vi "毕设初次修改版.vi"() -> ()   [LabVIEW 2018]
uses:
  <vilib>/addons/control/pid/pid.llb/PID (DBL).vi
  <vilib>/express/express arith-compare/Formula/XNode/ExpressFormulaBlockNode.xnode
  <vilib>/addons/control/pid/NI_PID_pid.lvlib
panel:
  out "密码文件路径":path
  out "操作人员0+密码":string[][](array[string])
  out "管理人员1+密码":string[][](array[string])
  out "用户名的顺序":u16
  out "用户类别":u8
  out "Error Out":errorcluster caption="错误输出"
  in  "Error In":errorcluster caption="错误输入"
  out "选项卡":T1(tab)
  in  "进入":bool
  in  "实验三界面":bool
  in  "其他界面":bool
  in  "实验二界面":bool
  in  "实验一界面":bool
  in  "提交界面":bool
  in  "公告栏":string[](array[string])=["欢迎您试用本实验平台", "本次的实验内容有", "1xxxxxxxx", "2cccccccc", "3dddddd", "4xxxxxxxx", "5vvvvvvvv"]
  in  "退出":bool
  out "图片":picture caption="新图片"
  in  "用户管理":bool
  out "当前用户类别":string
  out "当前用户名":string
  out "时间":string
  out "小卡":enum32{"1.1", "1.2"}(tab)
  in  "下页":bool
  out "过程变量和设定值":cluster{dbl, "SP：":dbl}(graph)
  out "操作变量":dbl(graph)
  out "MV：":dbl(slide) scale=-100.0..100.0
  in  "SP：":dbl(slide) min=0.0 max=0.0 scale=0.0..120.0
  out "PV：":dbl(slide) scale=0.0..120.0
  in  "PID增益设定":T2={"比例增益(Kc)"=1.0, "积分时间(Ti，分)"=0.002, "微分时间(Td，分)"=0.002} {"微分时间(Td，分)" format="%.3f"; "积分时间(Ti，分)" format="%.3f"; "比例增益(Kc)" format="%.3f"}
  in  "实验一开始":bool
  in  "实验一暂停":bool
  in  "返回 2":bool
  out "实验1图":dbl[](graph)
  in  "上页":bool
  out "动态性能指标显示":T3
  out "是否合格显示":T4
  out "尝试次数":string
  out "可否提交":bool
  in  "返回 3":bool
  out "上升时间":dbl
  out "调节时间":dbl
  out "超调量":dbl
  in  "实验二暂停":bool
  in  "实验二开始":bool
  in  "对象特性设置":cluster{"num":dbl[], "den":dbl[]}={"num"=[1.0], "den"=[0.02, 1.0]}
  in  "PID增益设置":cluster{"Kp":dbl, "Ki":dbl, "Kd":dbl}={"Kp"=1.5, "Ki"=0.35, "Kd"=1.0}
  out "XY图":cluster{dbl[], dbl[]}(graph)
  in  "SP":dbl(slide) min=0.0 max=0.0 scale=0.0..120.0
  in  "返回 4":bool
  in  "Word保存地址":path=path "F:/LabVIEW练习/毕设/实验报告.doc"
  in  "提交确定":bool
  in  "学号:":string
  in  "姓名:":string="小明"
  in  "ExcelS.path":path=path "F:/LabVIEW练习/毕设/实验成绩.xls" caption="Excel保存路径"
  in  "空白":bool
  in  "初始化":bool
  in  "返回":bool
  in  "Excel模板路径":path=path "F:/LabVIEW练习/毕设/实验成绩.xls"
  in  "Word模板路径":path=path "F:/LabVIEW练习/毕设/实验报告模板.doc"
  out "实验3图表":dbl(graph)
  in  "实验三暂停":bool
  in  "实验三开始":bool
  in  "返回 5":bool
  in  "Kp":dbl=30.0 format="%#_13g"
  out "source":string
  out "尝试次数":u32
  in  "超限累计":i32
  out "数组":dbl[](array[numeric])=[0.15946790534816901, 0.35556228083290553, 0.5907826417638008, 0.8494826417638008, 1.1081826417638008, 1.3668826417638007, 1.6255826417638006, 1.8842826417638006, 2.1429826417638007, 2.401682641763801, 2.660382641763801, 2.919082641763801, 3.1777826417638013, 3.4364826417638015, 3.6951826417638016, 3.9538826417638018, 4.2125826417638015, 4.471282641763802, 4.729982641763802, 4.988682641763802, 5.247382641763802, 5.506082641763802, 5.764782641763802, 6.0234826417638025, 6.282182641763803, 6.540882641763803, 6.799582641763803, 7.058282641763803, 7.316982641763803, 7.5756826417638035, 7.834382641763804, 8.093082641763804, 8.351782641763803, 8.610482641763802, 8.869182641763802, 9.1278826417638, 9.3865826417638, 9.6452826417638, 9.903982641763799, 10.162682641763798, 10.421382641763797, 10.680082641763796, 10.938782641763796, 11.197482641763795, 11.456182641763794, 11.714882641763793, 11.973582641763793, 12.232282641763792, 12.490982641763791, 12.74968264176379, 13.00838264176379, 13.267082641763789, 13.525782641763788, 13.784482641763788, 14.043182641763787, 14.301882641763786, 14.560582641763785, 14.819282641763785, 15.077982641763784, 15.336682641763783, 15.595382641763782, 15.854082641763782, 16.112782641763783, 16.371482641763784, 16.630182641763785, 16.888882641763786, 17.147582641763787, 17.406282641763788, 17.66498264176379, 17.92368264176379, 18.18238264176379, 18.441082641763792, 18.699782641763793, 18.958482641763794, 19.217182641763795, 19.475882641763796, 19.734582641763797, 19.9932826417638, 20.2519826417638, 20.5106826417638, 20.7693826417638, 21.028082641763802, 21.286782641763804, 21.545482641763805, 21.804182641763806, 22.062882641763807, 22.321582641763808, 22.58028264176381, 22.83898264176381, 23.09768264176381, 23.356382641763812, 23.615082641763813, 23.873782641763814, 24.132482641763815, 24.391182641763816, 24.649882641763817, 24.908582641763818, 25.16728264176382, 25.42598264176382, 25.68468264176382, 25.943382641763822, 26.202082641763823, 26.460782641763824, 26.719482641763825, 26.978182641763826, 27.236882641763827, 27.49558264176383, 27.75428264176383, 28.01298264176383, 28.27168264176383, 28.530382641763833, 28.789082641763834, 29.047782641763835, 29.306482641763836, 29.565182641763837, 29.823882641763838, 30.08258264176384, 30.34128264176384, 30.59998264176384, 30.858682641763842, 31.117382641763843, 31.376082641763844, 31.634782641763845, 31.893482641763846, 32.152182641763844, 32.41088264176384, 32.66958264176384, 32.928282641763836, 33.186982641763834, 33.44568264176383, 33.70438264176383, 33.963082641763826, 34.221782641763824, 34.48048264176382, 34.73918264176382, 34.997882641763816, 35.25658264176381, 35.51528264176381, 35.77372176165425, 36.031884459742486, 36.289771162313485, 36.54738216334767, 36.80471775760098, 37.061778239505244, 37.318522130243544, 37.57467358720941, 37.8299594264456, 38.084107940043786, 38.33686499688974, 38.587925999781845, 38.837015689907915, 39.08390098833731, 39.32828579607282, 39.56990831464298, 39.80852799499046, 40.04390159016064, 40.275777925533525, 40.503874950422215, 40.72793097876865, 40.94778181593828, 41.16322788169536, 41.3740472034328, 41.580023389427126, 41.78087973060037, 41.97645279482925, 42.166568681508785, 42.35103471778728, 42.52957941340393, 42.70208708634859, 42.86840732714809, 43.02827548540423, 43.18150954430742, 43.32806311134, 43.46781164646614, 43.600619222636375, 43.726357743660884, 43.84490694692867, 43.956154516980234, 44.05986646431542, 44.15606406402364, 44.24453639469577, 44.32519057948923, 44.39795443410196, 44.462764470554774, 44.51956602229976, 44.5684623722877, 44.60942425329443, 44.64227082069252, 44.666977641637374, 44.683534283119904, 44.69193920908696, 44.692359011378294, 44.68465028908381, 44.668999121914815, 44.64527563307593, 44.61352408042584, 44.57379545987751, 44.52614939302406, 44.47081710257968, 44.407867701626955, 44.3372216673248, 44.25897957356577, 44.17340367346343, 44.0804305099236, 43.98034675420013, 43.87326265304072, 43.75930728668722, 43.63846143518952, 43.511038790252734, 43.377022593732704, 43.23673818240778, 43.09033207622225, 42.93782851259838, 42.77956724262933, 42.615570642290564, 42.44618643585735, 42.271586813576505, 42.091838302223536, 41.90729733314443, 41.71802441898804, 41.52425881526584, 41.32633897695649, 41.12446160950261, 40.918741029655656, 40.70954089926177, 40.4969648106794, 40.281375841949064, 40.06298482798073, 39.84203160577297, 39.61875810290718, 39.39332769049512, 39.166094497507856, 38.937206459131936, 38.707011747084934, 38.47566953230472, 38.24346340376417, 38.01064870010497, 37.7774810808516, 37.54421607075162, 37.31114593136907, 37.07849129310784, 36.84650071747841, 36.615378575927984, 36.38537198581724, 36.156943040417275, 35.93015564000529, 35.70525048381508, 35.482464651506554, 35.26203247520919, 35.04418528714419, 34.82918977838842, 34.61728362150174, 34.40866418976721, 34.203545417677866, 34.002152710466156, 33.80468049370989, 33.611355630079316, 33.42235243373588, 33.237840660649525, 33.058071096130554, 32.88318656057269, 32.71334221077529, 32.548785239587595, 32.38970558748683, 32.23635039277429, 32.0887213027308, 31.94692772347299, 31.811109866020686, 31.681500382105583, 31.558141994624826, 31.441138071257893, 31.330710906159855, 31.226982177337977, 31.130051544807788, 31.03989192894575, 30.956574187060063, 30.880298416516695, 30.811016574667573, 30.748779172798816, 30.693770570174408, 30.64604383266606, 30.605500125335514, 30.57216235661245, 30.546191212341355, 30.52746301020953, 30.515979813151755, 30.511739148217686, 30.514730768837623, 30.525082405205367, 30.54262096493095, 30.567314262688704, 30.599121227790977, 30.63799326089107, 30.684022094229924, 30.737138109376353, 30.79712134083411, 30.864047204647928, 30.937674402846334, 31.01791864742922, 31.104680413124612, 31.197997533983642, 31.297601112667355, 31.403524770877823, 31.51548742435686, 31.633369889626856, 31.75717052786516, 31.886727545997974, 32.02188775690319, 32.16249207258547, 32.30824736260859, 32.45925547191968, 32.615179595589765, 32.77573670801291, 32.940882235017824, 33.110406544352976, 33.28411560358437, 33.46181107958789, 33.64318536552284, 33.82805847807178, 34.01632346763871, 34.20774500171118, 34.40210761886112, 34.59910568351407, 34.79863001296244, 35.00043309118822, 35.20421455937076, 35.409776861426906, 35.616895997678924, 35.82540967343328, 36.03500330478898, 36.245529997989294, 36.45673189274724, 36.66833177613277, 36.88016878368664, 37.09198479004521, 37.30354852280296, 37.514602306871495, 37.72494707482634, 37.93437652215988, 38.142624707699454, 38.349505294607624, 38.5547654289942, 38.758213276831206, 38.95961027411947, 39.15877000170116, 39.355468869927705, 39.54949168753746, 39.74066037677261, 39.92877582472998, 40.11361003289667, 40.29498171485171, 40.47268498177152, 40.64651067819616, 40.816326941874074, 40.98192711472907, 41.14317621204567, 41.29986838770229, 41.451821738844906, 41.5988799580375, 41.7409664432832, 41.87795719408764, 42.0097157520009, 42.13611165526278, 42.257020452567055, 42.372232010346224, 42.481617154649165, 42.585166458979025, 42.6826931531345, 42.774090098791774, 42.859376819902224, 42.938376129353465, 43.0110039302606, 43.0773083298165, 43.13700634690593, 43.19026686553209, 43.23706044447938, 43.27722730725126, 43.310855788692564, 43.33780207941015, 43.35817371768441, 43.37183675931807, 43.37878738416311, 43.379031648389216, 43.372714902851996, 43.35985733742113, 43.340486081998, 43.31463518904689, 43.28234558282003, 43.2436650014862, 43.198513698357374, 43.14695891512083, 43.08906997124019, 43.024922996561216, 42.95460080492671, 42.878324985411076, 42.79604942541201, 42.708016010792086, 42.61432063883826, 42.51494734919351, 42.41015434896103, 42.299927660461705, 42.184411727942404, 42.06386503485702, 41.938293151587985, 41.80785840805722, 41.672713132822174, 41.53312773424592, 41.389244209130915, 41.241117376020824, 41.08893540101152, 40.932975542979875, 40.77329393535387, 40.61018892311368, 40.44382249205406, 40.27428885036583, 40.10180013164225, 39.926634944570246, 39.74896521510243, 39.568986518363765, 39.38689637097467, 39.20289414894689, 39.017114489970886, 38.82984923352281, 38.641279065899965, 38.45160880070593, 38.2609929339156, 38.06966498568467, 37.87787826534298, 37.68577681806894]
  # "结果显示"
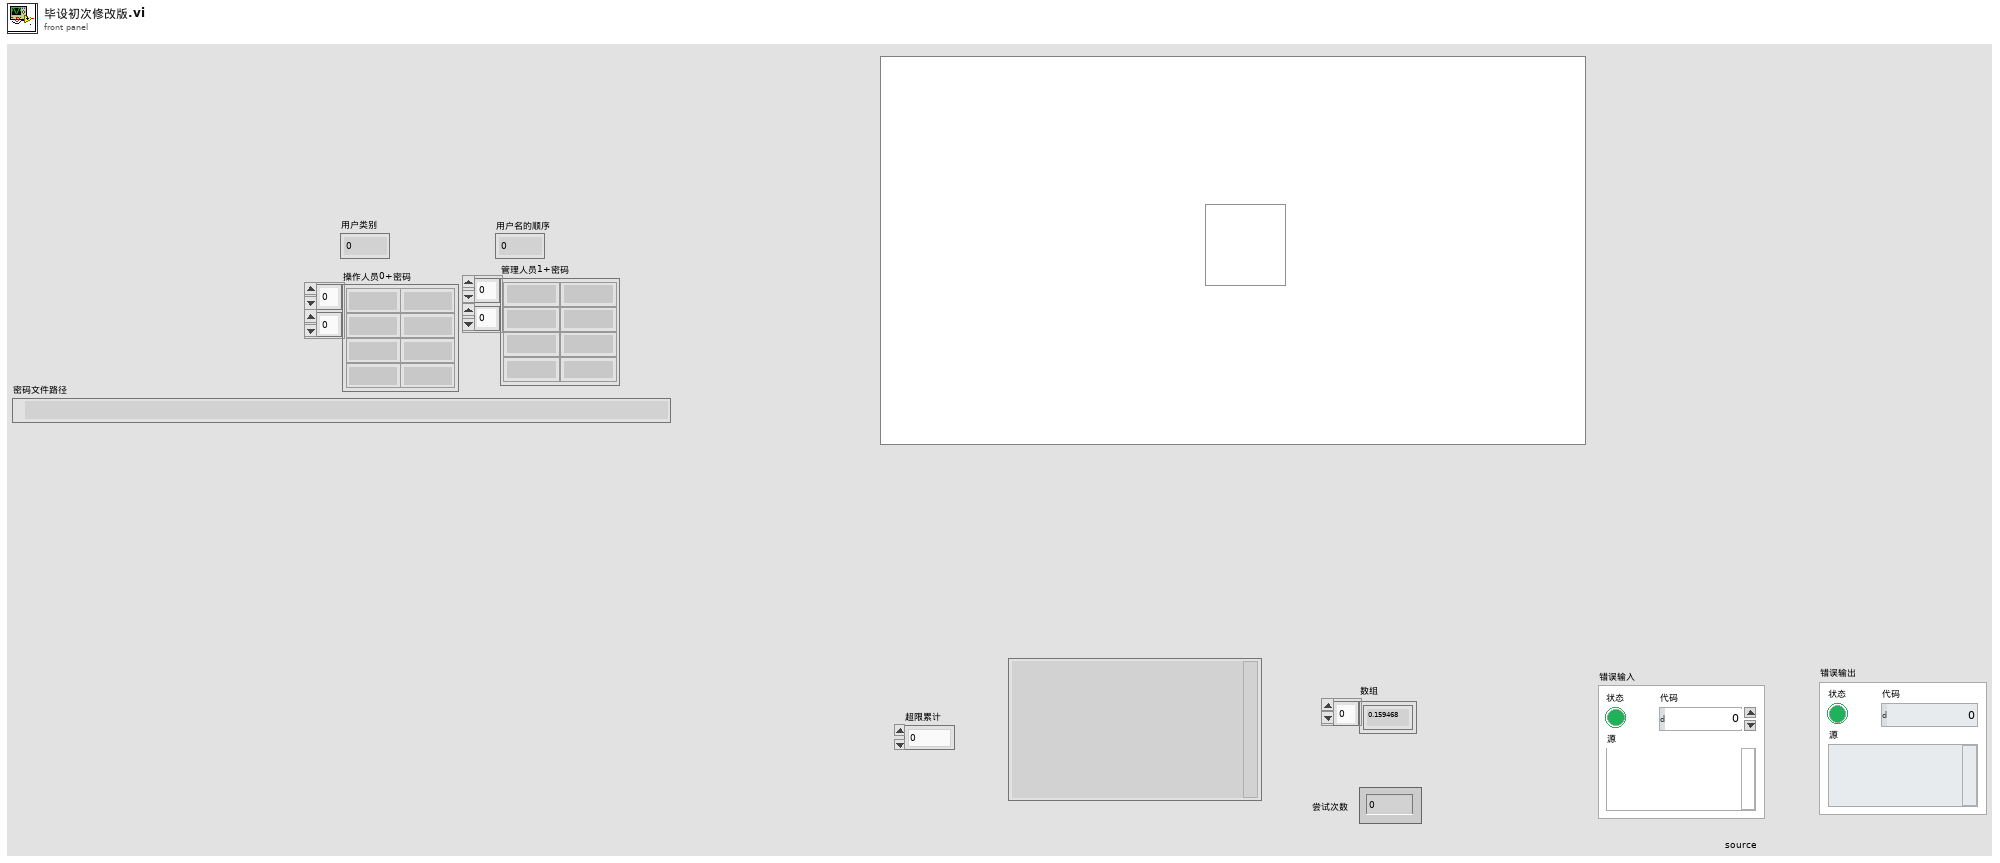
[diagram p1: front panel]
types:
  T1 = enum32{"登录", "公告", "实验1", "实验2", "提交", "其他", "实验3"}
  T2 = cluster{"比例增益(Kc)":dbl, "积分时间(Ti，分)":dbl, "微分时间(Td，分)":dbl}
  T3 = cluster{"超调量":string, "振荡频率":string, "调节时间":string, " 峰值时间":string, "阻尼比 ":string}
  T4 = cluster{"超调量":string, "振荡频率":string, "调节时间":string}
  T5 = typedef "全局事件选择.ctl" = enum16{"初始化", "等待操作", "空白", "退出", "进入", "提交确定", "返回主界面", "实验一界面", "实验二界面", "提交界面", "实验二开始", "实验一开始", "实验一暂停", "其他界面", "实验三界面", "实验三开始", "实验二暂停", "实验三暂停", "用户管理"}
  T6 = cluster{"操作人员0+密码":string[][], "管理人员1+密码":string[][]}
  T7 = enum32{"invalid app kind", "Development System", "Run Time System", "Student Edition", "Embedded LabVIEW", "Evaluation", "Custom"}
  T8 = cluster{"Excel模板路径":path, "Word模板路径":path, "ExcelS.path":path, "Word保存地址":path}
  T9 = cluster{"Font Name:":string, "Size":i16, "Strikeout?":bool, "Italic?":bool, bool, "Outline?":bool, "Shadow?":bool, "Bold?":bool}
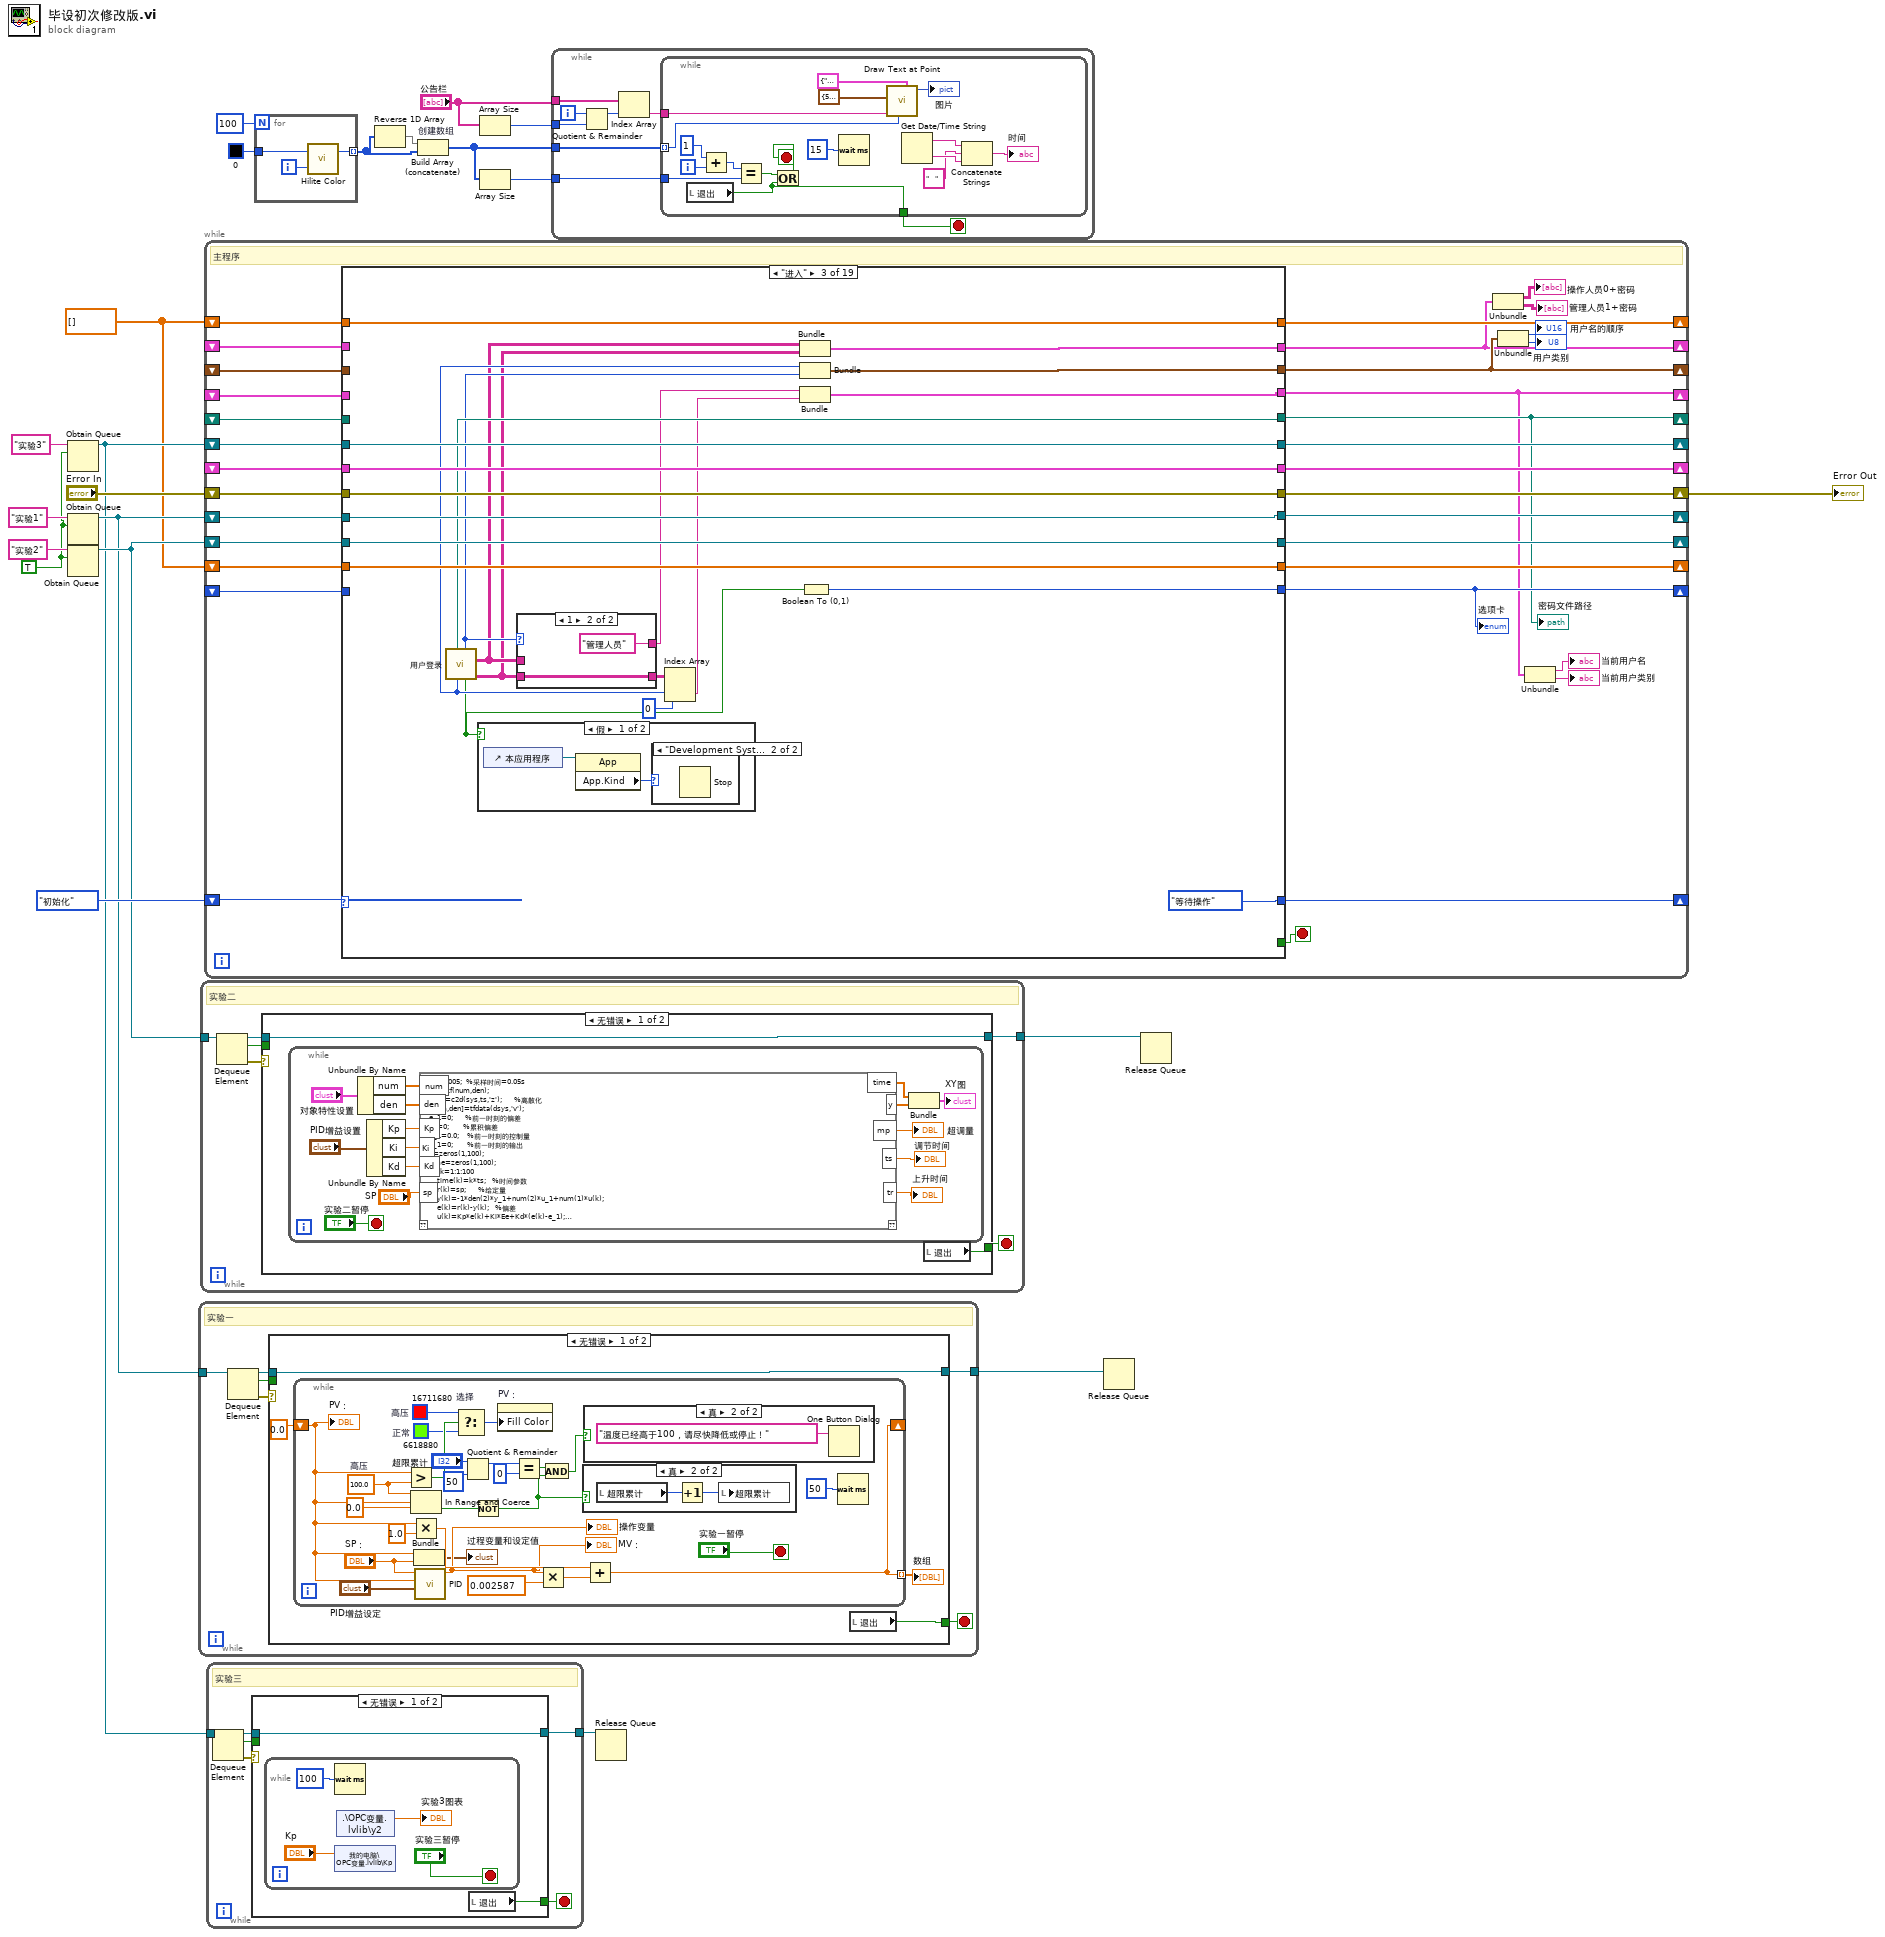
[diagram p0: block diagram]
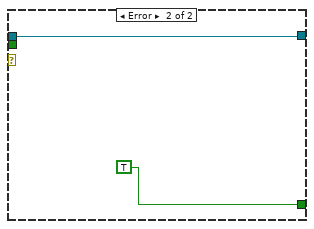
[diagram p2: hidden frame]
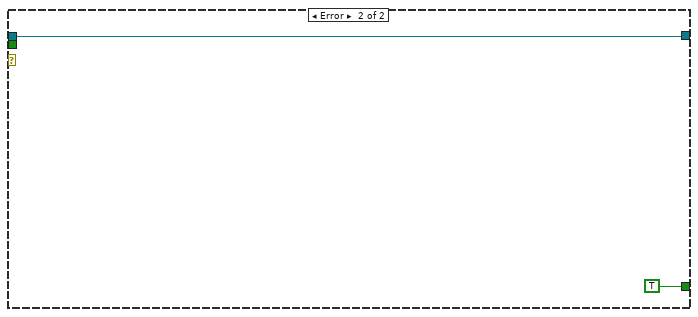
[diagram p5: hidden frame]
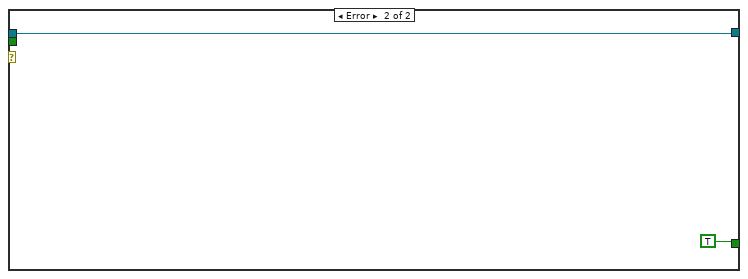
[diagram p6: hidden frame]
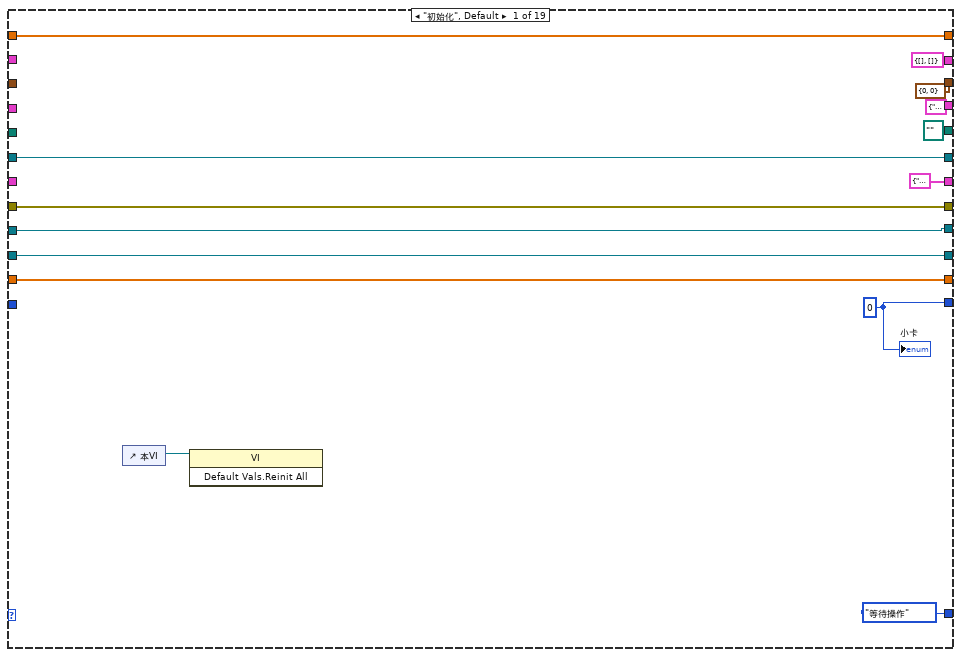
[diagram p7: hidden frame]
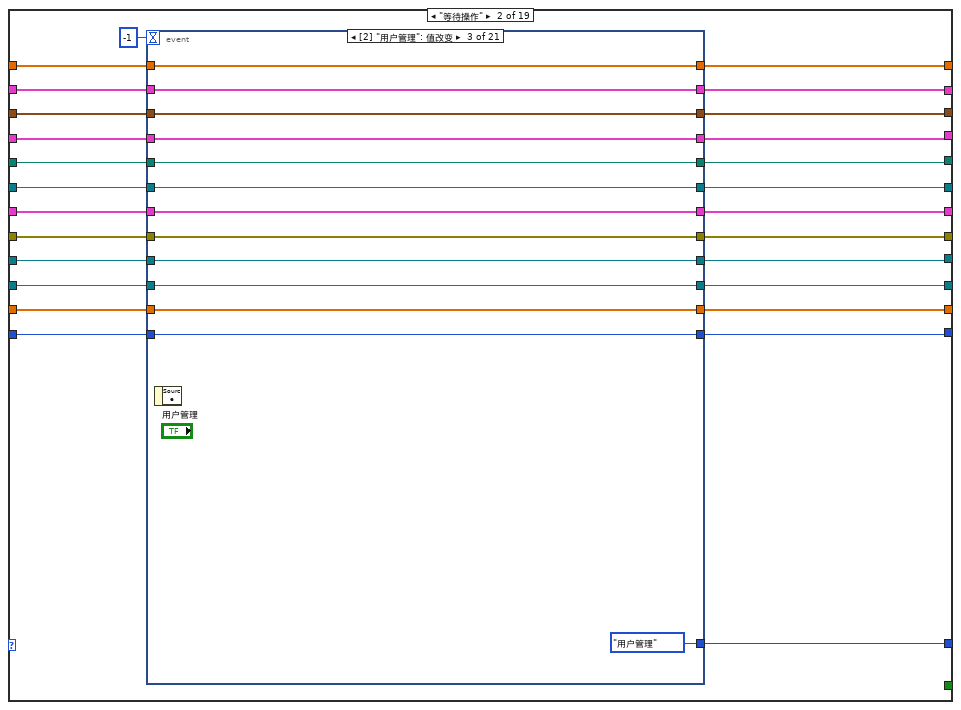
[diagram p8: hidden frame]
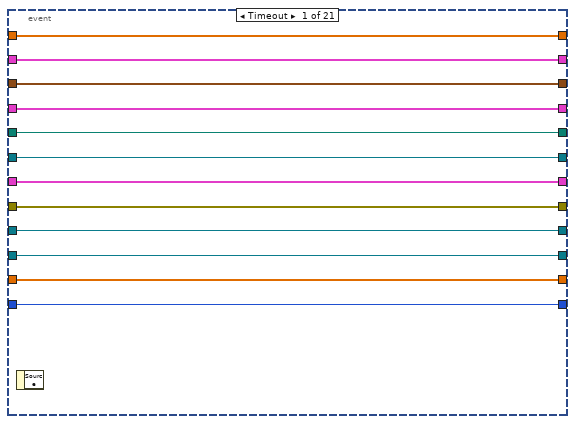
[diagram p9: hidden frame]
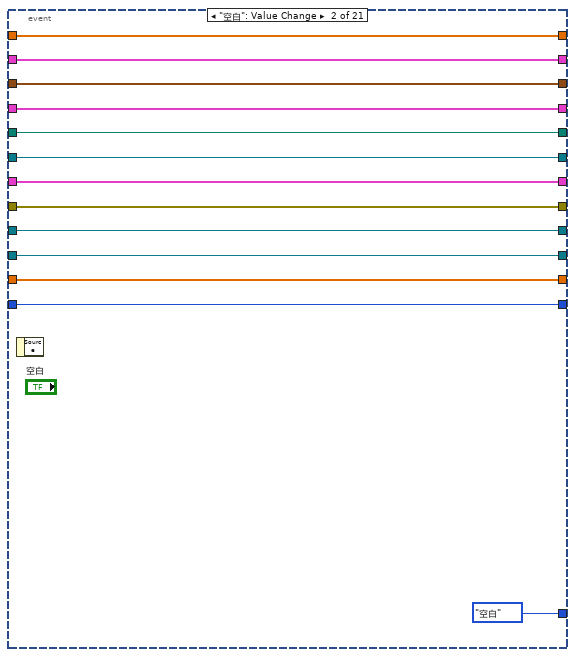
[diagram p10: hidden frame]
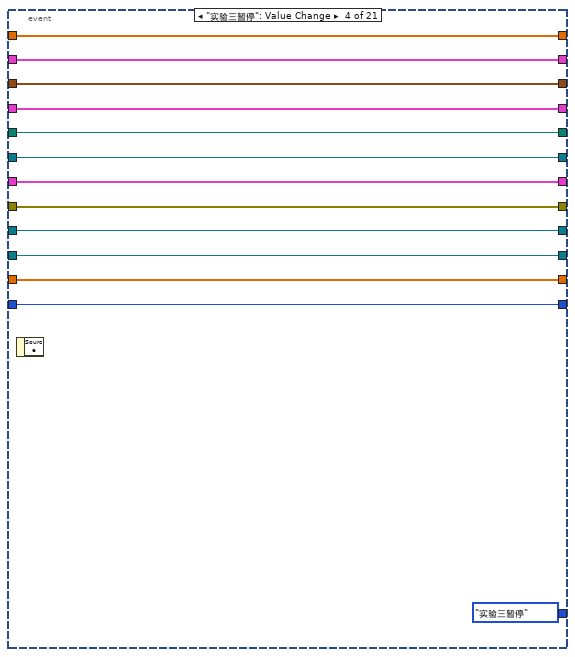
[diagram p11: hidden frame]
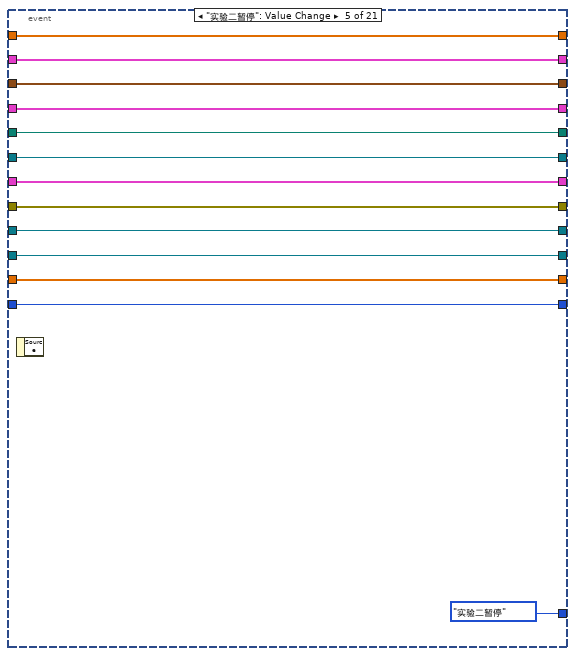
[diagram p12: hidden frame]
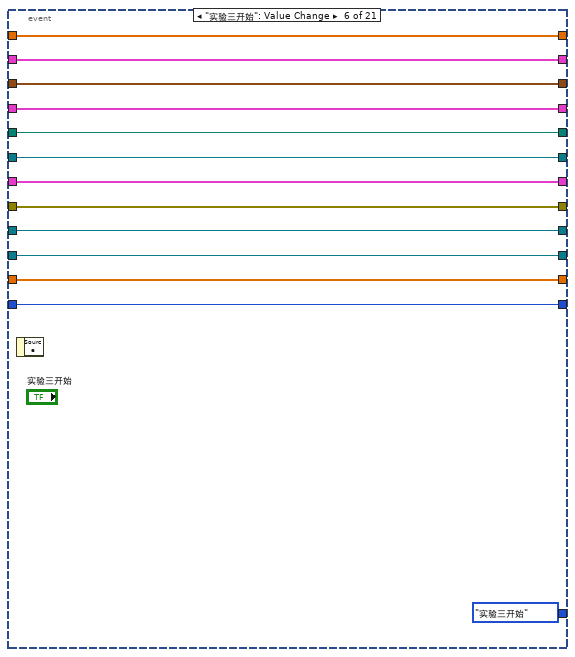
[diagram p13: hidden frame]
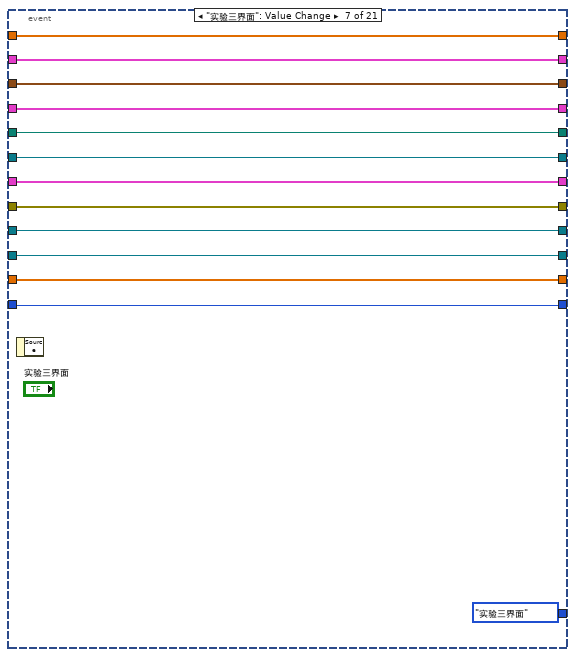
[diagram p14: hidden frame]
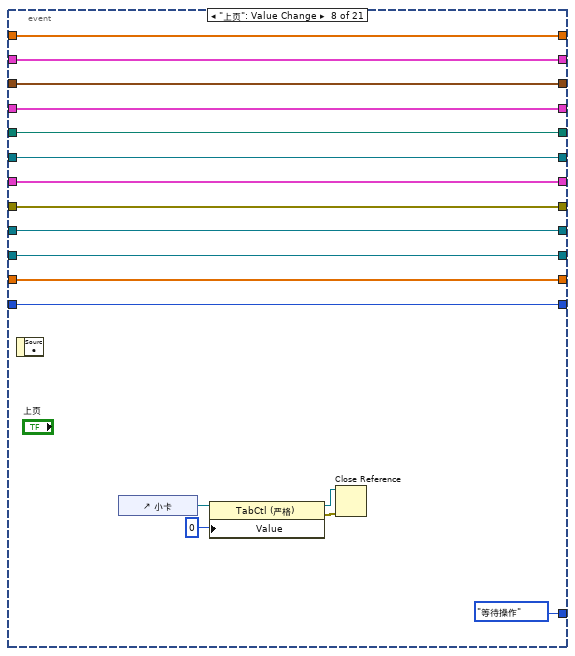
[diagram p15: hidden frame]
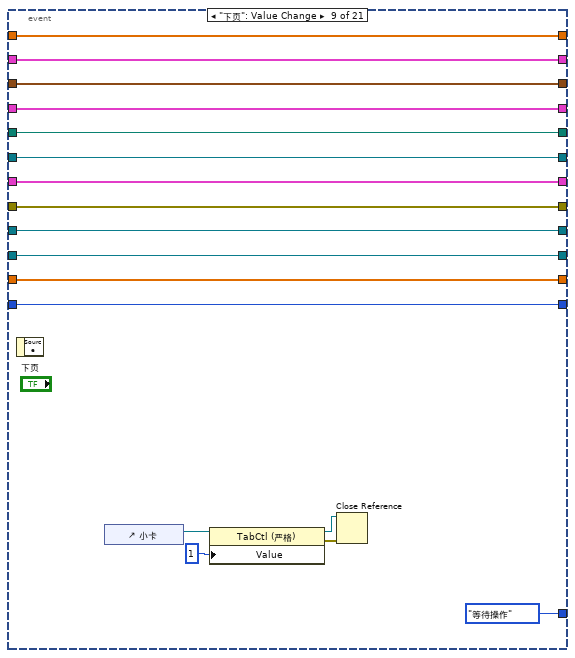
[diagram p16: hidden frame]
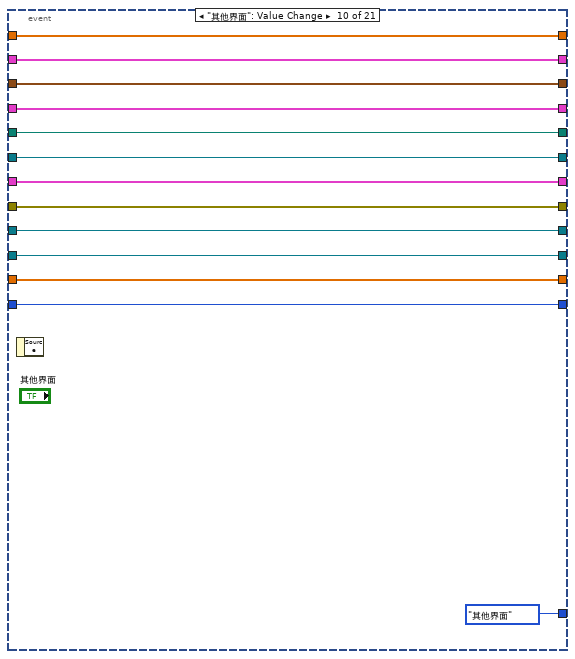
[diagram p17: hidden frame]
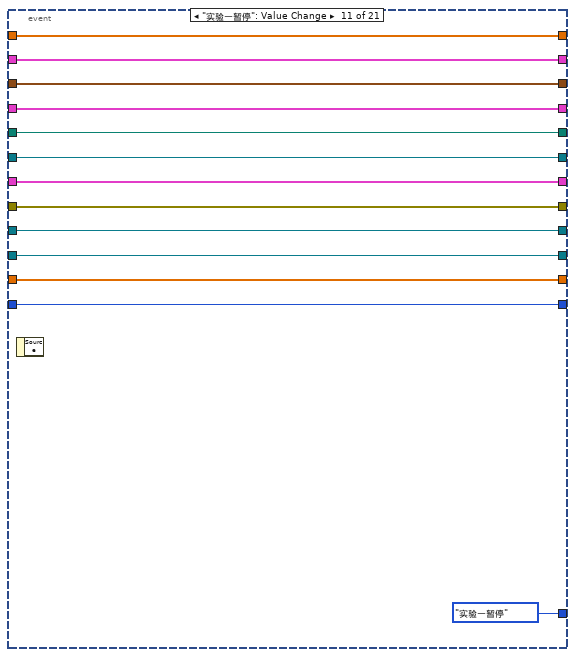
[diagram p18: hidden frame]
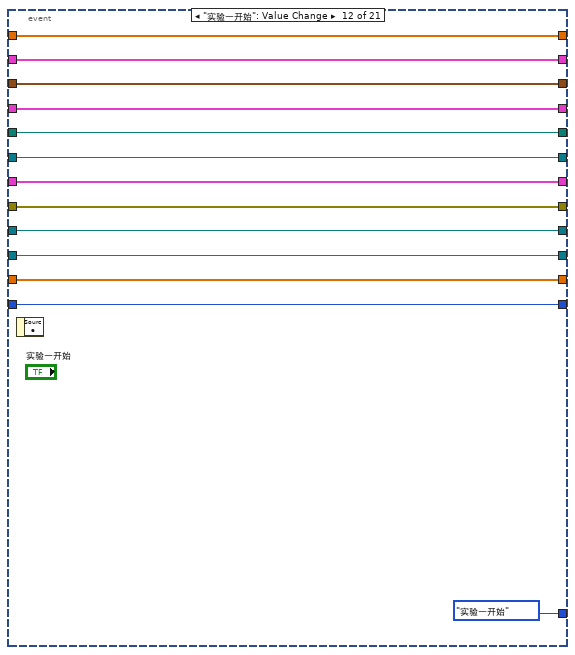
[diagram p19: hidden frame]
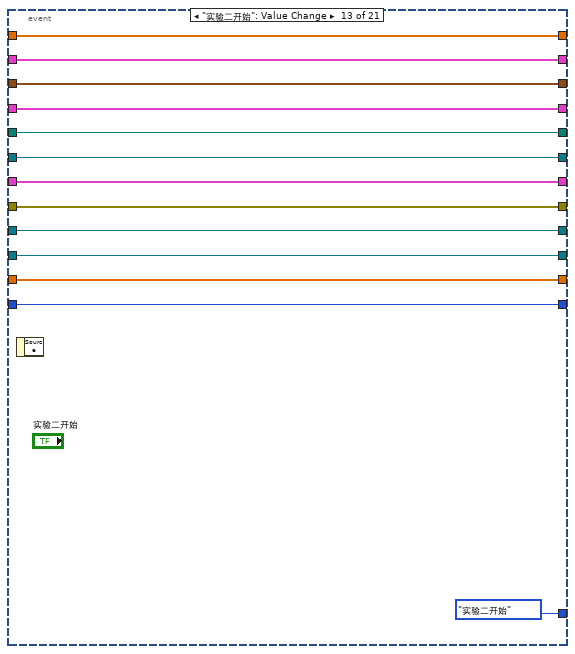
[diagram p20: hidden frame]
diagram:
  w11 = TRUE
  w1 = dbl[] []
  n1 = Obtain Queue(name (unnamed)="实验3" ("名称（未命名）"), element data type=w11) -> (queue out=w10:refnum<queue>)  [unwired: 3 in, 2 out]
  n2 = Obtain Queue(name (unnamed)="实验1" ("名称（未命名）"), element data type=w11) -> (queue out=w17:refnum<queue>)  [unwired: 3 in, 2 out]
  n3 = Obtain Queue(name (unnamed)="实验2" ("名称（未命名）"), element data type=w11) -> (queue out=w20:refnum<queue>)  [unwired: 3 in, 2 out]
  n4 = while {
    tunnel: w17 -> [w28]
    tunnel: [w23] -> w16
    stop <- w25 stop-if-true
    # "实验一"
    n5 = Dequeue Element(queue=w28) -> (queue out=w24:refnum<queue>, element=w26:bool, error out=w27:errorcluster)  [unwired: 2 in, 1 out]
    n6 = case shown="无错误" w27 {
      tunnel: w26 -> [_ _]
      tunnel: [w29 TRUE] -> w25
      tunnel: w24 -> [w32 w62]
      tunnel: [w32 w62] -> w23
      frame No Error {
        n7 = while {
          shift-right: [w50] -> _
          shift-left: 0.0 -> [w43]
          tunnel: [w50] -> w31 mode=indexing
          stop <- "实验一暂停" stop-if-true
          w45 = u32 6618880  # 正常
          w44 = u32 16711680  # 高压
          w46 = 100.0  # 高压
          n8 = Greater?(x=w43, y=w46) -> (0:w48:bool)
          n9 = In Range and Coerce ("判定范围并强制转换")(upper limit=w46, x=w43, lower limit=0.0 ("下限")) -> (In Range?=w49:bool)  [unwired: 1 out]
          n10 = Multiply(x=w43, y=1.0) -> (x*y=w55:dbl)
          n11 = Bundle(w43, "SP："="SP：") -> (→"过程变量和设定值":cluster{dbl, "SP：":dbl})  [unwired: 1 in]
          n12 = call-poly <vilib>:"PID.vi"("PID gains"="PID增益设定", "process variable"=w43, "setpoint"="SP：") -> ("output"=w53:dbl)  [unwired: 7 in, 1 out]
          "MV：" <- w53
          "操作变量" <- w53
          n13 = Select "选择"(t=w44, s=w48, f=w45) -> (s? t:f=w42:u32)
          n14 = Quotient & Remainder(x="超限累计", y=50) -> (x-y*floor(x/y)=w38:i32)  [unwired: 1 out]
          n15 = Not(x=w49) -> (.not. x?=w41:bool)
          n16 = property on="PV：" class="Slide (严格)"("Fill Color"=w42) -> ()  [unwired: 2 in, 2 out]
          n17 = Equal?(x=w38, y=0) -> (x = y?=w36:bool)
          n18 = Multiply(x=w53, y=0.002587) -> (x*y=w56:dbl)
          n19 = And(x=w36, y=w41) -> (x .and. y?=w35:bool)
          n20 = case shown="真" w41 {
            frame False {
            }
            frame True {
              n21 = local read "超限累计"() -> (w59:i32)
              n22 = Increment(x=w59) -> (x+1=w60:i32)
              n23 = local write "超限累计"(w60) -> ()
            }
          }
          n24 = case shown="真" w35 {
            frame False {
            }
            frame True {
              n25 = One Button Dialog ("单按钮对话框")(message="温度已经高于100，请尽快降低或停止！") -> ()  [unwired: 1 in, 1 out]
            }
          }
          n26 = Add(x=w55, y=w56) -> (x+y=w50:dbl)
          n27 = Wait (ms)(milliseconds to wait=50) -> ()  [unwired: 1 out]
          "PV：" <- w43
        }
        "数组" <- w31
        n28 = local read "退出"() -> (w29:bool)
      }
      frame Error {
      }
    }
  }
  n29 = while {
    tunnel: w20 -> [w69]
    tunnel: [w64] -> w19
    stop <- w66 stop-if-true
    # "实验二"
    n30 = Dequeue Element(queue=w69) -> (queue out=w65:refnum<queue>, element=w67:bool, error out=w68:errorcluster)  [unwired: 2 in, 1 out]
    n31 = case shown="无错误" w68 {
      tunnel: w67 -> [_ _]
      tunnel: [w70 TRUE] -> w66
      tunnel: w65 -> [w71 w87]
      tunnel: [w71 w87] -> w64
      frame No Error {
        n32 = while {
          stop <- "实验二暂停" stop-if-true
          n33 = Unbundle By Name("对象特性设置") -> ("num"=w79:dbl[], "den"=w78:dbl[])
          n34 = Unbundle By Name("PID增益设置") -> ("Kp"=w82:dbl, "Ki"=w81:dbl, "Kd"=w80:dbl)
          n35 = script code="ts=0.005;  %采样时间=0.05s\nsys=tf(num,den);   \ndsys=c2d(sys,ts,'z');      %离散化\n[num,den]=tfdata(dsys,'v');\ne_1=0;      %前一时刻的偏差      \nEe=0;       %累积偏差\nu_1=0.0;    %前一时刻的控制量\ny_1=0;       %前一时刻的输出\nu=zeros(1,100);\ntime=zeros(1,100);\nfor k=1:1:100\n    time(k)=k*ts;   %时间参数\n    r(k)=sp;      %给定量\n    y(k)=-1*den(2)*y_1+num(2)*u_1+num(1)*u(k);\n    e(k)=r(k)-y(k);   %偏差\n    u(k)=Kp*e(k)+Ki*Ee+Kd*(e(k)-e_1);   \n    Ee=Ee+e(k);    \n    u_1=u(k);    \n    y_1=y(k);    \n    e_1=e(k);\nend\nn=length(time);\n[ymax,ind]=max(y);\nyss=y(n);\ntp=time(ind);\nmp=100*(ymax-yss)/yss;\ny1=1.05*yss;\ny2=0.95*yss;\nk=n;\nwhile k>0\nk=k-1;\nif y(k)>=y1|y(k)<=y2;\nm=k;\nx=y(k);\nts=time(m);\nbreak;\nend\nend\nfor k=1:n\nif y(k)<=0.9*yss&y(k+1)>=0.9*yss\ntr=time(k);\nbreak\nend\nend"("Kp"=w82, "Ki"=w81, "Kd"=w80, "sp"="SP", "num"=w79, "den"=w78) -> ("time"=w85:dbl[], "y"=w84:dbl[], "mp"=→"超调量":dbl, "ts"=→"调节时间":dbl, "tr"=→"上升时间":dbl)  [unwired: 1 in, 1 out]
          n36 = Bundle(w85, w84) -> (→"XY图":cluster{dbl[], dbl[]})  [unwired: 1 in]
        }
        n37 = local read "退出"() -> (w70:bool)
      }
      frame Error {
      }
    }
  }
  n38 = while {
    shift-right: [w101] -> _
    shift-left: 全局事件选择."初始化" ("枚举") -> [w121]
    shift-right: [w108] -> _
    shift-left: w1 -> [w120]
    shift-right: [w91] -> _
    shift-left: _ -> [w119]
    shift-right: [w97] -> _
    shift-left: _ -> [w118]
    shift-right: [w94] -> _
    shift-left: _ -> [w117]
    shift-right: [w98] -> _
    shift-left: _ -> [w116]
    shift-right: [w107] -> _
    shift-left: w10 -> [w115]
    shift-right: [w106] -> _
    shift-left: _ -> [w114]
    shift-right: [w105] -> w15
    shift-left: "Error In" -> [w113]
    shift-right: [w104] -> _
    shift-left: w17 -> [w112]
    shift-right: [w103] -> _
    shift-left: w20 -> [w111]
    shift-right: [w102] -> _
    shift-left: w1 -> [w110]
    shift-right: [w99] -> _
    shift-left: _ -> [w109]
    stop <- w100 stop-if-true
    # "主程序"
    n39 = case shown="\"进入\"" w121 {
      tunnel: [w135 w149 w463 w482 w507 w526 w547 w631 w673 w690 w720 w737 w754 w787 w800 w827 w840 w853 w867] -> w108
      tunnel: w120 -> [w135 w161 w463 w482 w507 w526 w547 w631 w673 w690 w720 w737 w754 w787 w800 w827 w840 w853 w867]
      tunnel: [T6 {"操作人员0+密码"=[], "管理人员1+密码"=[]} w148 w446 w481 w497 w525 w546 w630 w672 w689 w719 w736 w753 w786 w799 w826 w839 w852 w866] -> w91
      tunnel: w119 -> [_ w160 _ w481 w497 w525 w546 w630 w672 w689 w719 w736 w753 w786 w799 w826 w839 w852 w866]
      tunnel: [cluster{"用户名的顺序out":u16, "用户类别_out":u8} {"用户名的顺序out"=0, "用户类别_out"=0} w147 w449 w480 w496 w524 w545 w629 w671 w688 w718 w735 w752 w785 w798 w825 w838 w851 w865] -> w97
      tunnel: w118 -> [_ w159 _ w480 w496 w524 w545 w629 w671 w688 w718 w735 w752 w785 w798 w825 w838 w851 w865]
      tunnel: [cluster{string, "类别":string} {"", "类别"=""} w146 w442 w479 w506 w523 w544 w628 w670 w687 w717 w734 w751 w784 w797 w824 w837 w850 w864] -> w94
      tunnel: w117 -> [_ w158 _ w479 w506 w523 w544 w628 w670 w687 w717 w734 w751 w784 w797 w824 w837 w850 w864]
      tunnel: [path "" ("密码文件路径") w145 w452 w478 w488 w522 w543 w627 w669 w686 w716 w733 w750 w783 w796 w823 w836 w849 w863] -> w98
      tunnel: w116 -> [_ w157 _ w478 w488 w522 w543 w627 w669 w686 w716 w733 w750 w783 w796 w823 w836 w849 w863]
      tunnel: [w134 w144 w462 w477 w505 w521 w542 w626 w668 w685 w715 w732 w739 w782 w795 w822 w835 w848 w862] -> w107
      tunnel: w115 -> [w134 w156 w462 w477 w505 w521 w542 w626 w668 w685 w715 w732 w742 w782 w795 w822 w835 w848 w862]
      tunnel: [cluster{string, string, string, string, string} {"", "", "", "", ""} w143 w461 w476 w504 w520 w541 w577 w667 w684 w714 w731 w749 w781 w794 w816 w834 w847 w861] -> w106
      tunnel: w114 -> [_ w155 w461 w476 w504 w520 w541 _ w667 w684 w714 w731 w749 w781 w794 w816 w834 w847 w861]
      tunnel: [w123 w142 w460 w475 w503 w519 w535 w625 w666 w674 w713 w730 w738 w780 w793 w810 w833 w846 w860] -> w105
      tunnel: w113 -> [w123 w154 w460 w475 w503 w519 w536 w625 w666 w677 w713 w730 w743 w780 w793 w811 w833 w846 w860]
      tunnel: [w133 w141 w459 w474 w502 w518 w531 w624 w665 w683 w712 w729 w748 w779 w792 w821 w832 w845 w859] -> w104
      tunnel: w112 -> [w133 w153 w459 w474 w502 w518 w533 w624 w665 w683 w712 w729 w748 w779 w792 w821 w832 w845 w859]
      tunnel: [w132 w140 w458 w473 w501 w517 w540 w623 w664 w675 w711 w728 w747 w778 w791 w820 w831 w844 w858] -> w103
      tunnel: w111 -> [w132 w152 w458 w473 w501 w517 w540 w623 w664 w679 w711 w728 w747 w778 w791 w820 w831 w844 w858]
      tunnel: [w125 w139 w456 w472 w500 w516 w539 w622 w663 w682 w710 w727 w746 w777 w790 w819 w830 w843 w857] -> w102
      tunnel: w110 -> [w125 w151 w456 w472 w500 w516 w539 w622 w663 w682 w710 w727 w746 w777 w790 w819 w830 w843 w857]
      tunnel: [w122 w138 w455 w471 w499 2 w538 w621 3 w681 w709 6 w745 w776 4 w818 5 1 w856] -> w99
      tunnel: w109 -> [_ w150 _ w471 w499 _ w538 w621 _ w681 w709 _ w745 w776 _ w818 _ _ w856]
      tunnel: [全局事件选择."等待操作" ("枚举") w136 全局事件选择."等待操作" ("枚举") 全局事件选择."等待操作" ("枚举") 全局事件选择."等待操作" ("枚举") 全局事件选择."等待操作" ("枚举") 全局事件选择."等待操作" ("枚举") 全局事件选择."等待操作" ("枚举") 全局事件选择."等待操作" ("枚举") 全局事件选择."等待操作" ("枚举") 全局事件选择."等待操作" ("枚举") 全局事件选择."等待操作" ("枚举") 全局事件选择."等待操作" ("枚举") 全局事件选择."等待操作" ("枚举") 全局事件选择."等待操作" ("枚举") 全局事件选择."等待操作" ("枚举") 全局事件选择."等待操作" ("枚举") 全局事件选择."等待操作" ("枚举") 全局事件选择."等待操作" ("枚举")] -> w101
      tunnel: [_ _ _ _ _ _ _ _ _ _ _ _ _ _ _ _ _ _ w854] -> w100
      frame "初始化", Default {
        w122 = 0
        n40 = control-ref of="本VI"() -> (w124:refnum<vi>)
        n41 = invoke class="VI" method="Default Vals.Reinit All"(reference=w124) -> ()  [unwired: 2 in, 3 out]
        "小卡" <- w122
      }
      frame "等待操作" {
        n42 = event shown="[2] \"用户管理\": 值改变" {
          selector: _ -> [_ _ _ _ _ _ _ _ _ _ _ _ _ _ _ _ _ _ _ _ _]
          dyn-events: _ -> [_ _ _ _ _ _ _ _ _ _ _ _ _ _ _ _ _ _ _ _ _]
          timeout: -1 -> [_ _ _ _ _ _ _ _ _ _ _ _ _ _ _ _ _ _ _ _ _]
          tunnel: w161 -> [w173 w186 w199 w212 w225 w238 w251 w268 w285 w298 w311 w324 w337 w350 w363 w376 w389 w402 w415 w428 w441]
          tunnel: [w173 w186 w199 w212 w225 w238 w251 w268 w285 w298 w311 w324 w337 w350 w363 w376 w389 w402 w415 w428 w441] -> w149
          tunnel: w160 -> [w172 w185 w198 w211 w224 w237 w250 w267 w284 w297 w310 w323 w336 w349 w362 w375 w388 w401 w414 w427 w440]
          tunnel: w159 -> [w171 w184 w197 w210 w223 w236 w249 w266 w283 w296 w309 w322 w335 w348 w361 w374 w387 w400 w413 w426 w439]
          tunnel: w158 -> [w170 w183 w196 w209 w222 w235 w248 w265 w282 w295 w308 w321 w334 w347 w360 w373 w386 w399 w412 w425 w438]
          tunnel: w157 -> [w169 w182 w195 w208 w221 w234 w247 w264 w281 w294 w307 w320 w333 w346 w359 w372 w385 w398 w411 w424 w437]
          tunnel: w156 -> [w168 w181 w194 w207 w220 w233 w246 w263 w280 w293 w306 w319 w332 w345 w358 w371 w384 w397 w410 w423 w436]
          tunnel: w155 -> [w167 w180 w193 w206 w219 w232 w245 w262 w279 w292 w305 w318 w331 w344 w357 w370 w383 w396 w409 w422 w435]
          tunnel: w154 -> [w166 w179 w192 w205 w218 w231 w244 w261 w278 w291 w304 w317 w330 w343 w356 w369 w382 w395 w408 w421 w434]
          tunnel: w153 -> [w165 w178 w191 w204 w217 w230 w243 w260 w277 w290 w303 w316 w329 w342 w355 w368 w381 w394 w407 w420 w433]
          tunnel: w152 -> [w164 w177 w190 w203 w216 w229 w242 w259 w276 w289 w302 w315 w328 w341 w354 w367 w380 w393 w406 w419 w432]
          tunnel: w151 -> [w163 w176 w189 w202 w215 w228 w241 w258 w275 w288 w301 w314 w327 w340 w353 w366 w379 w392 w405 w418 w431]
          tunnel: w150 -> [w162 w175 w188 w201 w214 w227 w239 w257 w274 w287 w300 w313 w326 w339 w352 w365 w378 w391 w404 w417 w430]
          tunnel: [w172 w185 w198 w211 w224 w237 w250 w267 w284 w297 w310 w323 w336 w349 w362 w375 w388 w401 w414 w427 w440] -> w148
          tunnel: [w171 w184 w197 w210 w223 w236 w249 w266 w283 w296 w309 w322 w335 w348 w361 w374 w387 w400 w413 w426 w439] -> w147
          tunnel: [w170 w183 w196 w209 w222 w235 w248 w265 w282 w295 w308 w321 w334 w347 w360 w373 w386 w399 w412 w425 w438] -> w146
          tunnel: [w169 w182 w195 w208 w221 w234 w247 w264 w281 w294 w307 w320 w333 w346 w359 w372 w385 w398 w411 w424 w437] -> w145
          tunnel: [w168 w181 w194 w207 w220 w233 w246 w263 w280 w293 w306 w319 w332 w345 w358 w371 w384 w397 w410 w423 w436] -> w144
          tunnel: [w167 w180 w193 w206 w219 w232 w245 w262 w279 w292 w305 w318 w331 w344 w357 w370 w383 w396 w409 w422 w435] -> w143
          tunnel: [w166 w179 w192 w205 w218 w231 w244 w261 w278 w291 w304 w317 w330 w343 w356 w369 w382 w395 w408 w421 w434] -> w142
          tunnel: [w165 w178 w191 w204 w217 w230 w243 w260 w277 w290 w303 w316 w329 w342 w355 w368 w381 w394 w407 w420 w433] -> w141
          tunnel: [w164 w177 w190 w203 w216 w229 w242 w259 w276 w289 w302 w315 w328 w341 w354 w367 w380 w393 w406 w419 w432] -> w140
          tunnel: [w163 w176 w189 w202 w215 w228 w241 w258 w275 w288 w301 w314 w327 w340 w353 w366 w379 w392 w405 w418 w431] -> w139
          tunnel: [w162 w175 w188 w201 w214 w227 w239 w257 w274 w287 w300 w313 w326 w339 w352 w365 w378 w391 w404 w417 w430] -> w138
          tunnel: [_ 全局事件选择."空白" ("枚举") 全局事件选择."用户管理" ("枚举") 全局事件选择."实验三暂停" ("枚举") 全局事件选择."实验二暂停" ("枚举") 全局事件选择."实验三开始" ("枚举") 全局事件选择."实验三界面" ("枚举") 全局事件选择."等待操作" ("枚举") 全局事件选择."等待操作" ("枚举") 全局事件选择."其他界面" ("枚举") 全局事件选择."实验一暂停" ("枚举") 全局事件选择."实验一开始" ("枚举") 全局事件选择."实验二开始" ("枚举") 全局事件选择."提交界面" ("枚举") 全局事件选择."实验一界面" ("枚举") 全局事件选择."实验二界面" ("枚举") 全局事件选择."返回主界面" ("枚举") 全局事件选择."提交确定" ("枚举") 全局事件选择."进入" ("枚举") 全局事件选择."初始化" ("枚举") 全局事件选择."退出" ("枚举")] -> w136
          event Timeout {
            n43 = event-data() -> ()  [unwired: 1 in, 1 out]
          }
          event "空白": Value Change {
            n44 = event-data() -> ()  [unwired: 1 in, 1 out]
          }
          event "用户管理": Value Change {
            n45 = event-data() -> ()  [unwired: 1 in, 1 out]
          }
          event "实验三暂停": Value Change {
            n46 = event-data() -> ()  [unwired: 1 in, 1 out]
          }
          event "实验二暂停": Value Change {
            n47 = event-data() -> ()  [unwired: 1 in, 1 out]
          }
          event "实验三开始": Value Change {
            n48 = event-data() -> ()  [unwired: 1 in, 1 out]
          }
          event "实验三界面": Value Change {
            n49 = event-data() -> ()  [unwired: 1 in, 1 out]
          }
          event "上页": Value Change {
            n50 = event-data() -> ()  [unwired: 1 in, 1 out]
            n51 = control-ref of="小卡"() -> (w252:refnum<vi>)
            n52 = property class="TabCtl (严格)"(reference=w252, "Value"=0) -> (reference out=w253:refnum<vi>, error out=w255:errorcluster)  [unwired: 1 in]
            n53 = Close Reference(reference=w253, error in (no error)=w255) -> ()  [unwired: 1 out]
          }
          event "下页": Value Change {
            n54 = event-data() -> ()  [unwired: 1 in, 1 out]
            n55 = control-ref of="小卡"() -> (w269:refnum<vi>)
            n56 = property class="TabCtl (严格)"(reference=w269, "Value"=1) -> (reference out=w272:refnum<vi>, error out=w271:errorcluster)  [unwired: 1 in]
            n57 = Close Reference(reference=w272, error in (no error)=w271) -> ()  [unwired: 1 out]
          }
          event "其他界面": Value Change {
            n58 = event-data() -> ()  [unwired: 1 in, 1 out]
          }
          event "实验一暂停": Value Change {
            n59 = event-data() -> ()  [unwired: 1 in, 1 out]
          }
          event "实验一开始": Value Change {
            n60 = event-data() -> ()  [unwired: 1 in, 1 out]
          }
          event "实验二开始": Value Change {
            n61 = event-data() -> ()  [unwired: 1 in, 1 out]
          }
          event "提交界面": Value Change {
            n62 = event-data() -> ()  [unwired: 1 in, 1 out]
          }
          event "实验一界面": Value Change {
            n63 = event-data() -> ()  [unwired: 1 in, 1 out]
          }
          event "实验二界面": Value Change {
            n64 = event-data() -> ()  [unwired: 1 in, 1 out]
          }
          event "返回", "返回 2", "返回 3", "返回 4", "返回 5": Value Change {
            n65 = event-data() -> ()  [unwired: 1 in, 1 out]
          }
          event "提交确定": Value Change {
            n66 = event-data() -> ()  [unwired: 1 in, 1 out]
          }
          event "进入": Value Change {
            n67 = event-data() -> ()  [unwired: 1 in, 2 out]
          }
          event "初始化": Value Change {
            n68 = event-data() -> ()  [unwired: 1 in, 1 out]
          }
          event "退出": Value Change {
            n69 = event-data() -> ()  [unwired: 1 in, 1 out]
          }
        }
      }
      frame "进入" {
        n70 = call "用户登录.vi"() -> ("管理人员1+密码"=w447:string[][], "操作人员0+密码"=w448:string[][], "T正常-F错误"=w445:bool, "用户类别_out"=w450:u8, "用户名的顺序out"=w451:u16, "密码文件路径"=w452:path)  [unwired: 4 in, 2 out]
        n71 = case shown="假" w445 {
          frame False {
            n72 = control-ref of="本应用程序"() -> (w468:refnum<vi>)
            n73 = property class="App"(reference=w468) -> ("App.Kind"=w469:T7)  [unwired: 1 in, 2 out]
            n74 = case shown="\"Development System\", 默认" w469 {
              frame "Run Time System" {
                n75 = Quit LabVIEW() -> ()  [unwired: 1 in]
              }
              frame "Development System", Default {
                n76 = Stop() -> ()  [unwired: 1 in]
              }
            }
          }
          frame True {
          }
        }
        n77 = case shown="1" w450 {
          tunnel: ["操作人员" "管理人员"] -> w444
          tunnel: w447 -> [_ w466]
          tunnel: [w464 w466] -> w454
          tunnel: w448 -> [w464 _]
          frame 0, Default {
          }
          frame 1 {
          }
        }
        n78 = Index Array(array=w454, index (row)=w451, index (col)=0 ("禁用的索引 (列)")) -> (element=w443:string)
        n79 = Bundle("操作人员0+密码"=w448, "管理人员1+密码"=w447) -> (w446:T6)  [unwired: 1 in]
        n80 = Bundle("用户名的顺序out"=w451, "用户类别_out"=w450) -> (w449:cluster{"用户名的顺序out":u16, "用户类别_out":u8})  [unwired: 1 in]
        n81 = Bundle(w444, "类别"=w443) -> (w442:cluster{string, "类别":string})  [unwired: 1 in]
        n82 = Boolean To (0,1)(Boolean=w445) -> (0, 1=w455:i16)
      }
      frame "空白" {
      }
      frame "用户管理" {
        n83 = Unbundle By Name(w496) -> ("用户类别_out"=w485:u8, "用户名的顺序out"=w484:u16)
        n84 = Unbundle By Name(w497) -> ("操作人员0+密码"=w487:string[][], "管理人员1+密码"=w486:string[][])
        n85 = call "用户管理.vi"("用户名的顺序"=w484, "用户类别"=w485, "管理人员1+密码"=w486, "操作人员0+密码"=w487, "密码文件路径"=w488) -> ("用户类别-out"=w494:u8, "管理人员1+密码-out"=w490:string[][], "操作人员0+密码-out"=w491:string[][], "用户名的顺序-out"=w489:u16)  [unwired: 2 in, 1 out]
        n86 = local write "操作人员0+密码"(w491) -> ()
        n87 = local write "管理人员1+密码"(w490) -> ()
        n88 = local write "用户名的顺序"(w489) -> ()
        n89 = case shown="0, 默认" w494 {
          tunnel: ["操作人员" "管理人员"] -> w493
          tunnel: w490 -> [_ w510]
          tunnel: [w508 w510] -> w495
          tunnel: w491 -> [w508 _]
          frame 0, Default {
          }
          frame 1 {
          }
        }
        n90 = local write "用户类别"(w494) -> ()
        n91 = local write "当前用户类别"(w493) -> ()
        n92 = Index Array(array=w495, index (row)=w489, index (col)=0 ("禁用的索引 (列)")) -> (element=w492:string)
        n93 = local write "当前用户名"(w492) -> ()
      }
      frame "实验一界面" {
        w513 = dbl[] [] ("历史数据")
        n94 = property on="操作变量" class="WFChart (严格)"("History Data"=w513) -> ()  [unwired: 2 in, 2 out]
        n95 = property on="过程变量和设定值" class="WFChart (严格)"("History Data"=cluster{dbl, "SP：":dbl}[] [] ("历史数据")) -> ()  [unwired: 2 in, 2 out]
        n96 = property on="实验1图" class="WFGraph (严格)"("Value"=w513) -> ()  [unwired: 2 in, 2 out]
      }
      frame "实验一开始" {
        n97 = control-ref of="超限累计"() -> (w528:refnum<vi>)
        n98 = control-ref of="尝试次数"() -> (w527:refnum<vi>)
        n99 = flat-sequence {
          tunnel: w527 -> [w563]
          tunnel: w528 -> [w559]
          tunnel: w536 -> [w555]
          tunnel: [w551] -> w534
          tunnel: w533 -> [w549]
          tunnel: [w549] -> w532
          tunnel: w534 -> [w566]
          tunnel: w532 -> [w568]
          tunnel: [w565] -> w530
          tunnel: [w567] -> w529
          tunnel: [w572] -> w531
          tunnel: [w573] -> w535
          tunnel: w530 -> [w573]
          tunnel: w529 -> [w572]
          frame #0 {
            w548 = dbl[] [] ("历史数据")
            n100 = property class="DigNum (严格)"(reference=w563, error in=w555) -> (reference out=w561:refnum<vi>, error out=w560:errorcluster, "Value"=w562:u32)
            n101 = property class="DigNum (严格)"(reference=w559, error in=w555, "Value"=-1) -> (reference out=w557:refnum<vi>, error out=w556:errorcluster)
            n102 = property on="操作变量" class="WFChart (严格)"("History Data"=w548) -> ()  [unwired: 2 in, 2 out]
            n103 = property on="过程变量和设定值" class="WFChart (严格)"("History Data"=cluster{dbl, "SP：":dbl}[] [] ("历史数据")) -> ()  [unwired: 2 in, 2 out]
            n104 = Increment(x=w562) -> (x+1=→"尝试次数":u32)
            n105 = Close Reference(reference=w561, error in (no error)=w560) -> (error out=w554:errorcluster)
            n106 = Close Reference(reference=w557, error in (no error)=w556) -> (error out=w553:errorcluster)
            n107 = property on="实验1图" class="WFGraph (严格)"("Value"=w548) -> ()  [unwired: 2 in, 2 out]
            n108 = Merge Errors(w554, w553) -> (w552:errorcluster)
            n109 = call <vilib>:"Clear Errors.vi"("error in (no error)"=w552) -> ("error out"=w551:errorcluster)  [unwired: 5 in, 1 out]
          }
          frame #1 {
            n110 = Enqueue Element(queue=w568, element=TRUE ("元素"), error in (no error)=w566) -> (queue out=w567:refnum<queue>, error out=w565:errorcluster)  [unwired: 1 in, 1 out]
          }
          frame #2 {
            w570 = 2
            n111 = control-ref of="实验一开始"() -> (w571:refnum<vi>)
            n112 = property class="Bool (严格)"(reference=w571, "DisabledEnum"=w570) -> ()  [unwired: 1 in, 2 out]
            n113 = property on="下页" class="Bool"("DisabledEnum"=w570) -> ()  [unwired: 2 in, 2 out]
            n114 = property on="返回 2" class="Bool"("DisabledEnum"=w570) -> ()  [unwired: 2 in, 2 out]
          }
        }
      }
      frame "实验一暂停" {
        w574 = 0
        w591 = "不合格"
        w590 = "合格"
        w585 = " s"
        w589 = 2
        n115 = control-ref of="实验一开始"() -> (w575:refnum<vi>)
        n116 = property on="尝试次数" class="DigNum (严格)"() -> ("Value"=w580:u32)  [unwired: 2 in, 2 out]
        n117 = property on="数组" class="Arr (严格)"() -> ("Value"=w578:dbl[])  [unwired: 2 in, 2 out]
        "实验1图" <- w578
        n118 = property class="Bool (严格)"(reference=w575, "DisabledEnum"=w574) -> ()  [unwired: 1 in, 2 out]
        n119 = property on="下页" class="Bool"("DisabledEnum"=w574) -> ()  [unwired: 2 in, 2 out]
        n120 = property on="返回 2" class="Bool"("DisabledEnum"=w574) -> ()  [unwired: 2 in, 2 out]
        n121 = Array Size(array=w578) -> (size(s)=w592:i32)
        n122 = Array Max & Min(array=w578) -> (max value=w615:dbl, max index (indices)=w613:i32)  [unwired: 2 out]
        n123 = Number To Decimal String(number=w580) -> (decimal integer string=→"尝试次数":string)  [unwired: 1 in]
        n124 = Decrement(x=w592) -> (x-1=w616:i32)
        n125 = Multiply(x=0.05, y=w613) -> (x*y=w610:dbl)
        n126 = Index Array(array=w578, index=w616) -> (element=w618:dbl)
        n127 = Subtract(x=w615, y=w618) -> (x-y=w617:dbl)
        n128 = Divide(x=w617, y=w618) -> (x/y=w611:dbl)
        n129 = xnode "公式"("X1"=w611) -> ("结果"=w619:dbl)  [unwired: 1 in, 1 out]
        n130 = Multiply(x=w611, y=100.0) -> (x*y=w602:dbl)
        n131 = xnode "公式 2"("X1"=w610, "X2"=w619) -> ("结果"=w600:dbl)  [unwired: 1 in, 1 out]
        n132 = xnode "公式 3"("X1"=w619, "X2"=w600) -> ("结果"=w601:dbl)  [unwired: 1 in, 1 out]
        n133 = Number To Fractional String(number=w602, precision (6)=w589) -> (F-format string=w614:string)  [unwired: 2 in]
        n134 = Number To Fractional String(number=w600, precision (6)=w589) -> (F-format string=w609:string)  [unwired: 2 in]
        n135 = Number To Fractional String(number=w601, precision (6)=w589) -> (F-format string=w608:string)  [unwired: 2 in]
        n136 = Number To Fractional String(number=w610, precision (6)=w589) -> (F-format string=w612:string)  [unwired: 2 in]
        n137 = Less Or Equal?(x=w602, y=10.0) -> (x <= y?=w594:bool)
        n138 = Less?(x=w601, y=15.0) -> (x < y?=w598:bool)
        n139 = Less?(x=w600, y=0.7) -> (x < y?=w596:bool)
        n140 = Number To Fractional String(number=w619, precision (6)=w589) -> (F-format string=w604:string)  [unwired: 2 in]
        n141 = Select(t=w590, s=w594, f=w591) -> (s? t:f=w593:string)
        n142 = Select(t=w590, s=w596, f=w591) -> (s? t:f=w595:string)
        n143 = Select(t=w590, s=w598, f=w591) -> (s? t:f=w597:string)
        n144 = Compound Arithmetic op=AND ("复合运算")(w594, w596, w598) -> (→"可否提交":bool)
        n145 = Concatenate Strings(w614, " %") -> (w607:string)
        n146 = Concatenate Strings(w609, " rad/s") -> (w605:string)
        n147 = Concatenate Strings(w608, w585) -> (w606:string)
        n148 = Concatenate Strings(w612, w585) -> (w603:string)
        n149 = Bundle(w593, w595, w597) -> (→"是否合格显示":cluster{string, string, string})  [unwired: 1 in]
        n150 = Bundle(w607, w605, w606, w603, w604) -> (w577:cluster{string, string, string, string, string})  [unwired: 1 in]
        "动态性能指标显示" <- w577
      }
      frame "实验二界面" {
        n151 = property on="实验二图" class="XYGraph (严格)"("Value"=cluster{dbl[], dbl[]} {[], []} ("XY图")) -> ()  [unwired: 2 in, 2 out]
      }
      frame "实验二开始" {
        n152 = flat-sequence {
          tunnel: w679 -> [w697]
          tunnel: [w697] -> w678
          tunnel: w677 -> [w696]
          tunnel: [w695] -> w676
          tunnel: w678 -> [w702]
          tunnel: w676 -> [w701]
          tunnel: [w700] -> w674
          tunnel: [w699] -> w675
          frame #0 {
            w691 = 3
            n153 = control-ref of="实验二开始"() -> (w692:refnum<vi>)
            n154 = property on="实验二图" class="XYGraph (严格)"(error in=w696, "Value"=cluster{dbl[], dbl[]} {[], []} ("XY图")) -> (error out=w695:errorcluster)  [unwired: 1 in, 1 out]
            n155 = property class="Bool"(reference=w692, "DisabledEnum"=w691) -> (reference out=w693:refnum<vi>, error out=w694:errorcluster)  [unwired: 1 in]
            n156 = property on="实验二开始" class="Bool"("DisabledEnum"=w691) -> ()  [unwired: 2 in, 2 out]
            n157 = property on="返回 3" class="Bool"("DisabledEnum"=w691) -> ()  [unwired: 2 in, 2 out]
            n158 = Close Reference(reference=w693, error in (no error)=w694) -> ()  [unwired: 1 out]
          }
          frame #1 {
            n159 = Enqueue Element(queue=w702, element=TRUE ("元素"), error in (no error)=w701) -> (queue out=w699:refnum<queue>, error out=w700:errorcluster)  [unwired: 1 in, 1 out]
          }
        }
      }
      frame "实验二暂停" {
        w704 = 0
        n160 = control-ref of="实验二开始"() -> (w705:refnum<vi>)
        n161 = property class="Bool"(reference=w705, "DisabledEnum"=w704) -> (reference out=w706:refnum<vi>, error out=w707:errorcluster)  [unwired: 1 in]
        n162 = property on="实验二开始" class="Bool"("DisabledEnum"=w704) -> ()  [unwired: 2 in, 2 out]
        n163 = property on="返回 3" class="Bool"("DisabledEnum"=w704) -> ()  [unwired: 2 in, 2 out]
        n164 = Close Reference(reference=w706, error in (no error)=w707) -> ()  [unwired: 1 out]
      }
      frame "实验三界面" {
        n165 = control-ref of="实验3图表"() -> (w722:refnum<vi>)
        n166 = property class="WFChart (严格)"(reference=w722, "History Data"=dbl[] [] ("历史数据")) -> (reference out=w724:refnum<vi>, error out=w723:errorcluster)  [unwired: 1 in]
        n167 = Close Reference(reference=w724, error in (no error)=w723) -> ()  [unwired: 1 out]
      }
      frame "实验三开始" {
        n168 = flat-sequence {
          tunnel: w743 -> [w762]
          tunnel: w742 -> [w761]
          tunnel: [w761] -> w741
          tunnel: [w760] -> w740
          tunnel: w741 -> [w769]
          tunnel: w740 -> [w768]
          tunnel: [w767] -> w738
          tunnel: [w766] -> w739
          frame #0 {
            w755 = 3
            n169 = control-ref of="实验三图表"() -> (w757:refnum<vi>)
            n170 = control-ref of="实验三开始"() -> (w765:refnum<vi>)
            n171 = property class="WFChart (严格)"(reference=w757, "History Data"=dbl[] [] ("历史数据")) -> (reference out=w759:refnum<vi>, error out=w758:errorcluster)  [unwired: 1 in]
            n172 = property class="Bool"(reference=w765, error in=w762, "DisabledEnum"=w755) -> (reference out=w763:refnum<vi>, error out=w764:errorcluster)
            n173 = property on="实验三开始" class="Bool"("DisabledEnum"=w755) -> ()  [unwired: 2 in, 2 out]
            n174 = property on="返回 5" class="Bool"("DisabledEnum"=w755) -> ()  [unwired: 2 in, 2 out]
            n175 = Close Reference(reference=w763, error in (no error)=w764) -> (error out=w760:errorcluster)
            n176 = Close Reference(reference=w759, error in (no error)=w758) -> ()  [unwired: 1 out]
          }
          frame #1 {
            n177 = Enqueue Element(queue=w769, element=TRUE ("元素"), error in (no error)=w768) -> (queue out=w766:refnum<queue>, error out=w767:errorcluster)  [unwired: 1 in, 1 out]
          }
        }
      }
      frame "实验三暂停" {
        w771 = 0
        n178 = control-ref of="实验三开始"() -> (w774:refnum<vi>)
        n179 = property class="Bool"(reference=w774, "DisabledEnum"=w771) -> (reference out=w772:refnum<vi>, error out=w773:errorcluster)  [unwired: 1 in]
        n180 = property on="实验三开始" class="Bool"("DisabledEnum"=w771) -> ()  [unwired: 2 in, 2 out]
        n181 = property on="返回 5" class="Bool"("DisabledEnum"=w771) -> ()  [unwired: 2 in, 2 out]
        n182 = Close Reference(reference=w772, error in (no error)=w773) -> ()  [unwired: 1 out]
      }
      frame "提交界面" {
      }
      frame "提交确定" {
        n183 = control-ref of="尝试次数"() -> (w809:refnum<vi>)
        n184 = property class="Str"(reference=w809, error in=w811) -> (reference out=w814:refnum<vi>, error out=w813:errorcluster, "Value"=w815:string)
        n185 = Close Reference(reference=w814, error in (no error)=w813) -> (error out=w812:errorcluster)
        n186 = control-ref of="实验1图"() -> (w801:refnum<vi>)
        n187 = Bundle("Excel模板路径"="Excel模板路径", "Word模板路径"="Word模板路径", "ExcelS.path"="ExcelS.path", "Word保存地址"="Word保存地址") -> (w806:T8)  [unwired: 1 in]
        n188 = call "报表.vi"("姓名:"="姓名:", "尝试次数"=w815, "学号:"="学号:", "Error In"=w812, "path"=w806, "动态性能指标"=w816, "WFGraph引用句柄"=w801) -> ("Error Out"=w810:errorcluster)  [unwired: 4 in]
      }
      frame "其他界面" {
      }
      frame "返回主界面" {
      }
      frame "退出" {
        w854 = TRUE ("停止？(T)")
        n189 = Stop(stop? (T)=w854) -> ()
      }
    }
    "选项卡" <- w99
    "密码文件路径" <- w98
    n190 = Unbundle(w91) -> ("操作人员0+密码"=→"操作人员0+密码":string[][], "管理人员1+密码"=→"管理人员1+密码":string[][])
    n191 = Unbundle(w97) -> ("用户名的顺序out"=→"用户名的顺序":u16, "用户类别_out"=→"用户类别":u8)
    n192 = Unbundle(w94) -> (→"当前用户名":string, "类别"=→"当前用户类别":string)
  }
  "Error Out" <- w15
  n193 = while {
    tunnel: w10 -> [w873]
    tunnel: [w868] -> w13
    stop <- w870 stop-if-true
    # "实验三"
    n194 = Dequeue Element(queue=w873) -> (queue out=w869:refnum<queue>, element=w871:bool, error out=w872:errorcluster)  [unwired: 2 in, 1 out]
    n195 = case shown="无错误" w872 {
      tunnel: w871 -> [_ _]
      tunnel: [w874 TRUE] -> w870
      tunnel: w869 -> [w875 w880]
      tunnel: [w875 w880] -> w868
      frame No Error {
        n196 = while {
          stop <- "实验三暂停" stop-if-true
          n197 = Wait (ms)(milliseconds to wait=u32 100 ("毫秒计时值")) -> ()  [unwired: 1 out]
          n198 = shared-variable "我的电脑\\OPC变量.lvlib\\Kp"("Kp") -> ()  [unwired: 1 in, 1 out]
          n199 = shared-variable ".\\OPC变量.lvlib\\y2"() -> (→"实验3图表":dbl)  [unwired: 1 in, 1 out]
        }
        n200 = local read "退出"() -> (w874:bool)
      }
      frame Error {
      }
    }
  }
  n201 = for {
    N: 100 -> [_]
    tunnel: u32 0 ("Color In") -> [w884]
    tunnel: [w882] -> w5 mode=indexing
    i -> [w883]
    n202 = call <vilib>:"Hilite Color.vi"("Percentage(30)"=w883, "Color In"=w884) -> ("Hilite"=w882:u32)  [unwired: 1 out]
  }
  n203 = Reverse 1D Array(array=w5) -> (reversed array=w6:u32[])
  n204 = Build Array (concatenate) "创建数组"(w6, w5) -> (w4:u32[])
  n205 = Array Size(array="公告栏") -> (size(s)=w7:i32)
  n206 = Array Size(array=w4) -> (size(s)=w3:i32)
  n207 = while {
    tunnel: "公告栏" -> [w892]
    tunnel: w7 -> [w890]
    tunnel: w4 -> [w887]
    tunnel: w3 -> [w886]
    i -> [w891]
    stop <- w885 stop-if-true
    n208 = Quotient & Remainder(x=w891, y=w890) -> (x-y*floor(x/y)=w889:i32)  [unwired: 1 out]
    n209 = Index Array(array=w892, index=w889) -> (element=w888:string)
    n210 = while {
      tunnel: w888 -> [w908]
      tunnel: w887 -> [w906] mode=indexing
      tunnel: w886 -> [w903]
      tunnel: [w899] -> w885
      i -> [w901]
      stop <- w897 stop-if-true
      n211 = local read "退出"() -> (w899:bool)
      n212 = Add(x=1, y=w901) -> (x+y=w902:i32)
      n213 = Equal?(x=w902, y=w903) -> (x = y?=w898:bool)
      n214 = Or(x=w898, y=w899) -> (x .or. y?=w897:bool)
      n215 = Wait (ms)(milliseconds to wait=u32 15 ("等待时间（毫秒）")) -> ()  [unwired: 1 out]
      n216 = call <vilib>:"Draw Text at Point.vi"("[user-specified font]"=T9 {"Font Name:"="应用程序字体", "Size"=28, "Strikeout?"=FALSE, "Italic?"=FALSE, TRUE, "Outline?"=FALSE, "Shadow?"=FALSE, "Bold?"=FALSE}, "text color(black)"=w906, "text"=w908, "origin"=cluster{"x":i16, "y":i16} {"x"=50, "y"=20}) -> ("new picture"=→"图片":picture)  [unwired: 6 in, 1 out]
      n217 = Get Date/Time String() -> (date string=w896:string, time string=w895:string)  [unwired: 3 in]
      n218 = Concatenate Strings(w896, "   ", w895) -> (→"时间":string)
    }
  }
  n219 = Release Queue(queue=w13) -> ()  [unwired: 2 in, 3 out]
  n220 = Release Queue(queue=w16) -> ()  [unwired: 2 in, 3 out]
  n221 = Release Queue(queue=w19) -> ()  [unwired: 2 in, 3 out]
